vi "DataTargetsGLOBAL (1).vi"() -> ()   [LabVIEW 2017]
panel:
  in  "Braking - PSI Target":dbl=5.0
  in  "Pushing - PRIMARY Time Target (s)":dbl=10.0
  in  "Pressure Limit - Magnetic Braking (PSI)":dbl=70.0
  in  "Fault - Automatic Timeout":i64=300
  in  "Braking - Time Target(s)":dbl=5.0
  in  "Pressure Limit - Suspension (PSI)":dbl=70.0
  in  "Braking - Acceleration Target (m/s2)":dbl=-0.5
  in  "Coast - Stopping Position Target (m)":dbl=1400.0
  in  "Coast - Brake Time Target (s)":dbl=5.0
  in  "Ready - Piezo Target (V)":dbl=1.8
  in  "Ready - Acceleration Target (m/s2)":dbl=0.5
  # "When making changes,\nEdit -> Make Current Values Default"
  # "Data >="
  # "Data >="
  # "Data >="
  # "Data >="
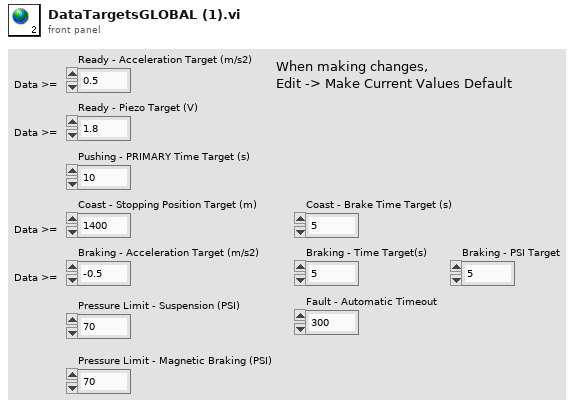
[diagram p1: front panel]
diagram:
